vi "svfa_Check Waveform Parameter Continuity (Nx1) [Dual FFT].vi"(0 "stimulus signal X [EUx]":waveform(dbl), 1 "restart averaging (F)":bool, 5 "response signals Y [EUy]":waveform(dbl)[](array[waveform]), 7 "checks for channel parameter change":T1, 9 "checks for multichannel parameters":T2, 11 "error in":errorcluster) -> (4 "dup stimulus signal X [EUx]":waveform(dbl), 6 "dup response signals Y [EUy]":waveform(dbl)[](array[waveform]), 8 "waveform parameter changed":bool, 10 "multichannel parameter changed":bool, 15 "error out":errorcluster)   [LabVIEW 2017]
uses:
  <vilib>/addons/_NISVFA/_Shared subVIs/Common/svc_Check for Waveform Parameter Continuity (no state).vi
  <vilib>/addons/_NISVFA/_Shared subVIs/Common/svc_Get SV Channel Info.vi
  <vilib>/addons/_NISVFA/_Shared subVIs/Common/svc_Engineering Units to Unit Label.vi
  <vilib>/addons/_NISVFA/_Shared subVIs/Common/svc_Unit Label to Engineering Units.vi
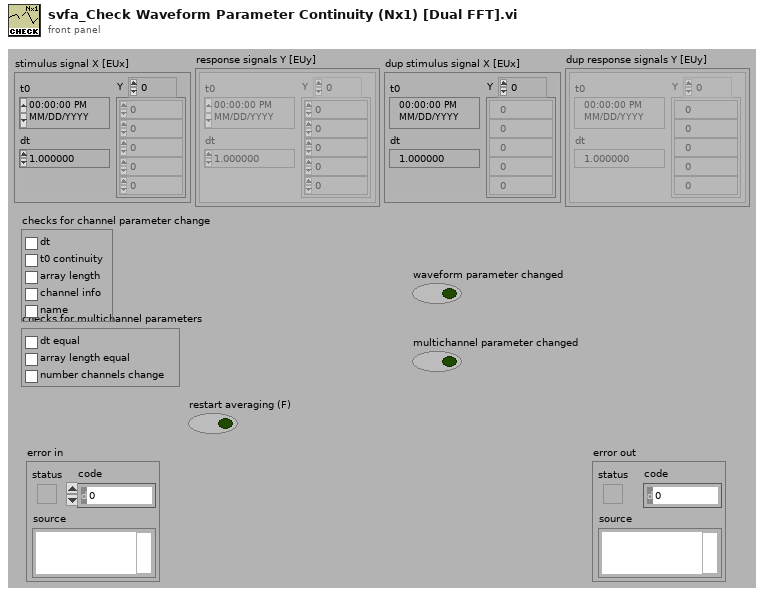
[diagram p1: front panel]
types:
  T1 = cluster{"dt":bool, "t0 continuity":bool, "array length":bool, "channel info":bool, "name":bool}
  T2 = cluster{"dt equal":bool, "array length equal":bool, "number channels change":bool}
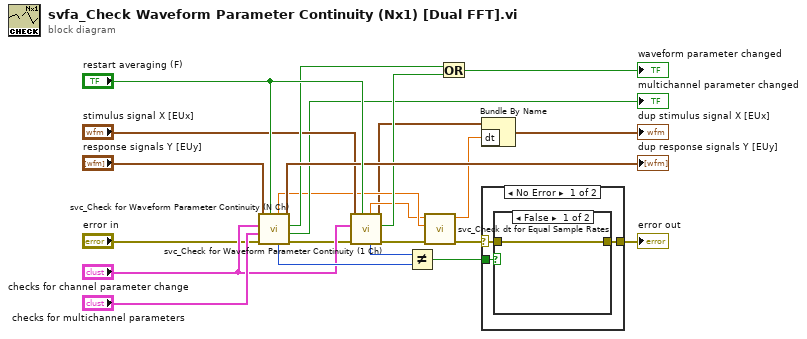
[diagram p0: block diagram]
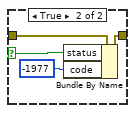
[diagram p2: hidden frame]
diagram:
  n1 = call <vilib>:"svc_Check for Waveform Parameter Continuity (N Ch).vi"("restart averaging (F)"="restart averaging (F)", "error in (no error)"="error in", "checks for multichannel parameters"="checks for multichannel parameters", "checks for channel parameter change"="checks for channel parameter change", "scaled signal(s)"="response signals Y [EUy]") -> ("error out"=w19:errorcluster, "multichannel parameter changed"=→"multichannel parameter changed":bool, "waveform parameter changed"=w14:bool, "dup scaled signal(s)"=→"dup response signals Y [EUy]":waveform(dbl)[], "array length"=w23:i32, "dt"=w8:dbl)  [unwired: 1 out]
  n2 = call <vilib>:"svc_Check for Waveform Parameter Continuity (1 Ch).vi"("restart averaging (F)"="restart averaging (F)", "error in (no error)"=w19, "checks for channel parameter change"="checks for channel parameter change", "scaled signal [EU]"="stimulus signal X [EUx]") -> ("error out"=w6:errorcluster, "waveform parameter changed"=w15:bool, "dup scaled signal [EU]"=w3:waveform(dbl), "array length"=w22:i32, "dt"=w7:dbl)  [unwired: 2 in, 1 out]
  n3 = Not Equal?(x=w22, y=w23) -> (x != y?=w4:bool)
  n4 = call <vilib>:"svc_Check dt for Equal Sample Rates.vi"("error in (no error)"=w6, "dt Y"=w8, "dt X"=w7) -> ("error out"=w9:errorcluster, "dt Y"=w1:dbl)  [unwired: 7 in]
  n5 = Or(x=w14, y=w15) -> (x .or. y?=→"waveform parameter changed":bool)
  n6 = Bundle By Name ("Build Waveform")(cluster=w3, "dt"=w1) -> (→"dup stimulus signal X [EUx]":waveform(dbl))
  n7 = case shown="No Error" w9 {
    selector: w9 -> [w25 w32]
    tunnel: w4 -> [w26 _]
    tunnel: [w24 w32] -> w5
    frame No Error {
      n8 = case shown="False" w26 {
        selector: w26 -> [_ w29]
        tunnel: [w27 w31] -> w24
        tunnel: w25 -> [w27 w28]
        frame False {
        }
        frame True {
          n9 = Bundle By Name(cluster=w28, "status"=w29, "code"=-1977) -> (w31:errorcluster)
        }
      }
    }
    frame Error {
    }
  }
  "error out" <- w5
